vi "Test Button.vi"(1 "ButtonProfile":i32[](array[numeric]), 2 "Buttons":T2, 3 "Button Type":T1(ring)=enum."Fire") -> (0 "Pressed?":bool)   [LabVIEW 2013]
uses:
  <vilib>/Rock Robotics/WPI/Joystick/WPI_JoystickButtonState.ctl
panel:
  # "Rob Stolarz was here\n\nLove you too\n\n2013-2014"
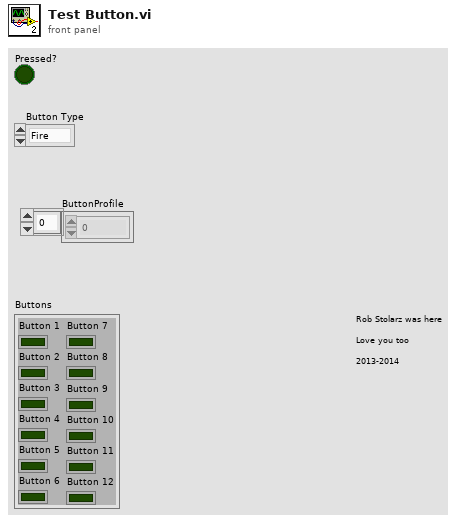
[diagram p1: front panel]
types:
  T1 = enum8{"Backward Spin WOT", "Forward Spin WOT", "Disengage WOT", "Engage WOT", "Kiddy Control", "Fire", "Override Finger"}
  T2 = typedef "WPI_JoystickButtonState.ctl" = cluster{"Button 1":bool, "Button 2":bool, "Button 3":bool, "Button 4":bool, "Button 5":bool, "Button 6":bool, "Button 7":bool, "Button 8":bool, "Button 9":bool, "Button 10":bool, "Button 11":bool, "Button 12":bool}
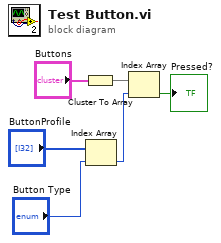
[diagram p0: block diagram]
diagram:
  n1 = Cluster To Array(cluster="Buttons") -> (array=w6:bool[])
  n2 = Index Array(array="ButtonProfile", index="Button Type") -> (element=w2:i32)
  n3 = Index Array(array=w6, index=w2) -> (element=→"Pressed?":bool)
